vi "Controller.vi"(0 "User Event in":refnum<user-event>, 1 "State":refnum<queue>, 3 "error in (state)":errorcluster) -> ()   [LabVIEW 2018]
uses:
  Desktop/StateMachineTest/2/Messages.ctl
  TimeCluster.ctl
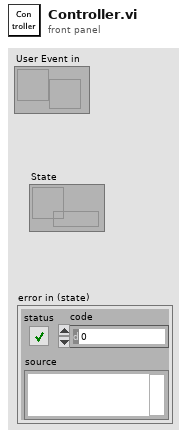
[diagram p1: front panel]
types:
  T1 = enum16{"On", "Off", "Preparation", "WaitTimer", "Ready"}
  T2 = typedef "TimeCluster.ctl" = cluster{"run":bool, "destroy":bool, "Elapsed time":i32, "WaitTime":i32, "Ticktime":i32}
  T3 = cluster{"Message":string, "Temp":i32, "Stato":enum16{"On", "Off", "Preparation", "WaitTimer", "Ready"}}
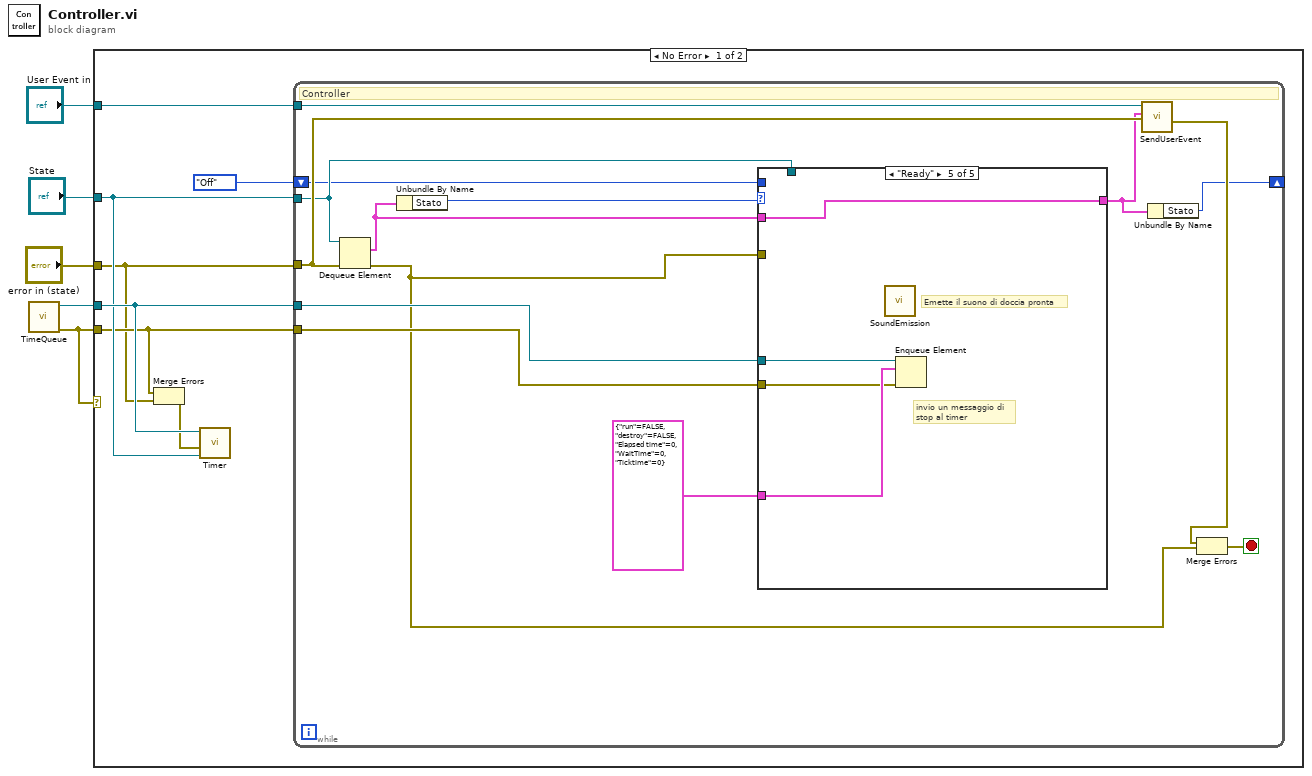
[diagram p0: block diagram]
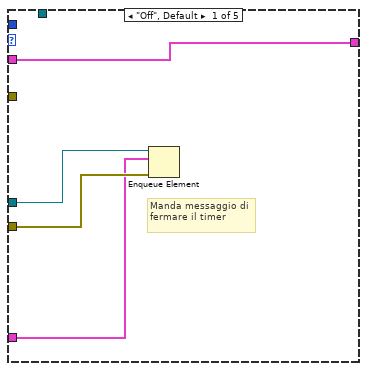
[diagram p2: hidden frame]
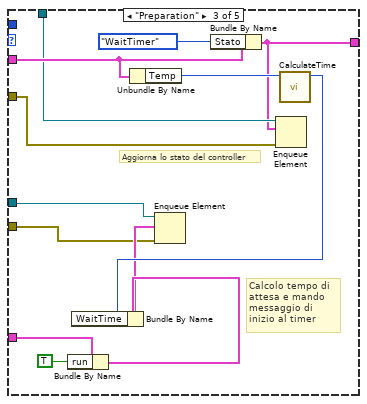
[diagram p4: hidden frame]
diagram:
  n1 = call "TimeQueue.vi"() -> ("error out"=w1:errorcluster, "Queue out"=w4:refnum<queue>)  [unwired: 10 in]
  n2 = case shown="No Error" w1 {
    tunnel: "User Event in" -> [w12 _]
    tunnel: w4 -> [w10 _]
    tunnel: "State" -> [w9 _]
    tunnel: w1 -> [w8 _]
    tunnel: "error in (state)" -> [w7 _]
    frame No Error {
      n3 = Merge Errors(w8, w7) -> (w6:errorcluster)
      n4 = call "Timer.vi"("State"=w9, "error in"=w6, "TimeQueue"=w10) -> ()  [unwired: 9 in]
      n5 = while {
        tunnel: w9 -> [w18]
        tunnel: w12 -> [w17]
        tunnel: w7 -> [w26]
        tunnel: w10 -> [w21]
        tunnel: w8 -> [w20]
        shift-right: [w14] -> _
        shift-left: T1."Off" -> [w13]
        stop <- w25 stop-if-true
        # "Controller"
        n6 = Dequeue Element(queue=w18, error in (no error)=w26) -> (element=w24:T3, error out=w16:errorcluster)  [unwired: 1 in, 2 out]
        n7 = Unbundle By Name(w24) -> ("Stato"=w19:T1)
        n8 = case shown="\"Ready\"" w19 {
          tunnel: [w30 w31 w34 w45 w46] -> w15
          tunnel: w24 -> [w30 w31 w37 w45 w46]
          tunnel: w20 -> [w28 _ w33 _ w47]
          tunnel: w21 -> [w29 _ w43 _ w49]
          tunnel: T2 {"run"=FALSE, "destroy"=FALSE, "Elapsed time"=0, "WaitTime"=0, "Ticktime"=0} -> [w27 _ w42 _ w48]
          tunnel: w18 -> [_ _ w35 _ _]
          tunnel: w16 -> [_ _ w32 _ _]
          tunnel: w13 -> [_ _ _ _ _]
          frame "Off", Default {
            # "Manda messaggio di fermare il timer"
            n9 = Enqueue Element(queue=w29, element=w27, error in (no error)=w28) -> ()  [unwired: 1 in, 3 out]
          }
          frame "On" {
            # "Stato di accensione, si attendono comandi dall'utente"
          }
          frame "Preparation" {
            # "Aggiorna lo stato del controller"
            # "Calcolo tempo di attesa e mando messaggio di inizio al timer"
            n10 = Bundle By Name(cluster=w42, "run"=TRUE) -> (w40:T2)
            n11 = Unbundle By Name(w37) -> ("Temp"=w38:i32)
            n12 = Bundle By Name(cluster=w37, "Stato"=T1."WaitTimer") -> (w34:T3)
            n13 = Enqueue Element(queue=w35, element=w34, error in (no error)=w32) -> ()  [unwired: 1 in, 3 out]
            n14 = call "CalculateTime.vi"("Temperatura"=w38) -> ("Tempo"=w44:i32)  [unwired: 10 in]
            n15 = Bundle By Name(cluster=w40, "WaitTime"=w44) -> (w39:T2)
            n16 = Enqueue Element(queue=w43, element=w39, error in (no error)=w33) -> ()  [unwired: 1 in, 3 out]
          }
          frame "WaitTimer" {
            # "Stato di attesa, in questo stato si attende il ready dal timer"
          }
          frame "Ready" {
            # "Emette il suono di doccia pronta"
            # "invio un messaggio di \nstop al timer"
            n17 = call "SoundEmission.vi"() -> ()  [unwired: 12 in]
            n18 = Enqueue Element(queue=w49, element=w48, error in (no error)=w47) -> ()  [unwired: 1 in, 3 out]
          }
        }
        n19 = call "SendUserEvent.vi"("error in (no error)"=w26, "Message Cluster"=w15, "User Event in"=w17) -> ("error out"=w22:errorcluster)  [unwired: 8 in]
        n20 = Unbundle By Name(w15) -> ("Stato"=w14:T1)
        n21 = Merge Errors(w22, w16) -> (w25:errorcluster)
      }
    }
    frame Error {
    }
  }
